vi "handle absolute files.vi"(8 "error in":errorcluster, 10 "absolute files":path[](array[path]), 11 "destination directory":path) -> (0 "error out":errorcluster)   [LabVIEW 2014]
uses:
  absolute file spec.ctl
  <vilib>/Utility/xml.llb/Write to XML File(string).vi
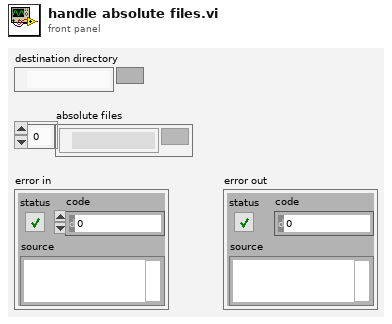
[diagram p1: front panel]
types:
  T1 = typedef "absolute file spec.ctl" = cluster{"name":string, "absolute path":path}
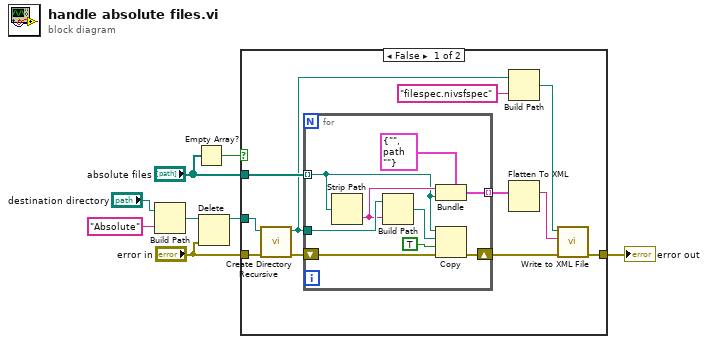
[diagram p0: block diagram]
diagram:
  n1 = Build Path(base path="destination directory", name or relative path="Absolute") -> (appended path=w3:path)
  n2 = Empty Array?(array="absolute files") -> (empty?=w6:bool)
  n3 = Delete(path (use dialog)=w3, error in="error in") -> (deleted path=w1:path)  [unwired: 3 in, 2 out]
  n4 = case shown="False" w6 {
    tunnel: [w19 w29] -> w8
    tunnel: w1 -> [w10 _]
    tunnel: "error in" -> [w13 w29]
    tunnel: "absolute files" -> [w12 _]
    frame False {
      n5 = call <vilib>:"Create Directory Recursive.vi"("error in (no error)"=w13, "directory"=w10) -> ("error out"=w11:errorcluster, "directory copy"=w9:path)  [unwired: 3 in, 1 out]
      n6 = for {
        shift-right: [w26] -> w16
        shift-left: w11 -> [w28]
        tunnel: w12 -> [w23] mode=indexing
        tunnel: w9 -> [w27]
        tunnel: [w22] -> w18 mode=indexing
        n7 = Strip Path(path=w23) -> (name=w24:string)  [unwired: 1 out]
        n8 = Build Path(base path=w27, name or relative path=w24) -> (appended path=w25:path)
        n9 = Bundle(cluster=T1 {"name"="", "absolute path"=path ""}, "name"=w24, "absolute path"=w23) -> (w22:T1)
        n10 = Copy(8:w28, 9:TRUE ("overwrite (F)"), 10:w25, 11:w23) -> (0:w26:errorcluster)  [unwired: 1 in, 2 out]
      }
      n11 = Build Path(base path=w9, name or relative path="filespec.nivsfspec") -> (appended path=w15:path)
      n12 = Flatten To XML(anything=w18) -> (xml string=w17:string)
      n13 = call-poly <vilib>:"Write to XML File.vi"("error in (no error)"=w16, "XML Input"=w17, "XML File Path"=w15) -> ("error out"=w19:errorcluster)  [unwired: 6 in, 2 out]
    }
    frame True {
    }
  }
  "error out" <- w8
